vi "XY2.vi"() -> (3 "XY Graph":cluster{"X":dbl, "Y":dbl}[](graph))   [LabVIEW 2023]
panel:
  in  "error constant 2":errorcluster
  out "error constant":errorcluster
  in  "XY Graph 2":cluster{"X":dbl, "Y":dbl}[](graph)
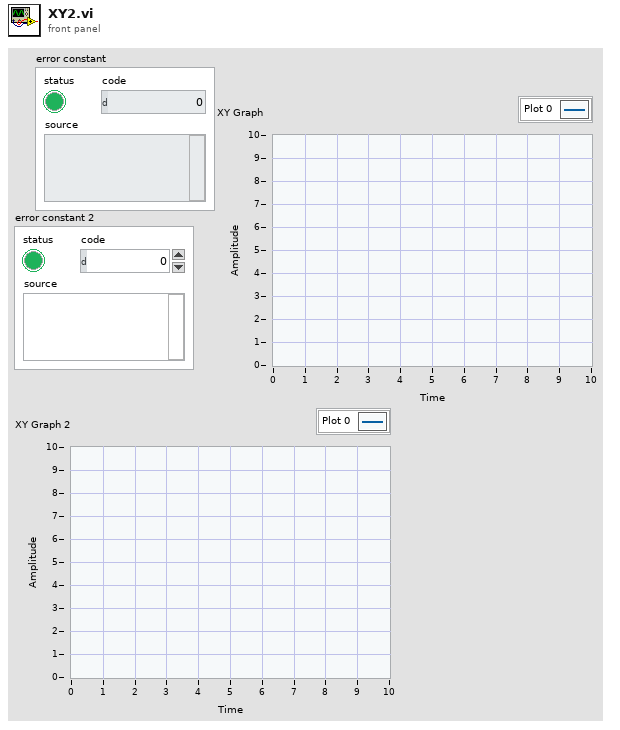
[diagram p1: front panel]
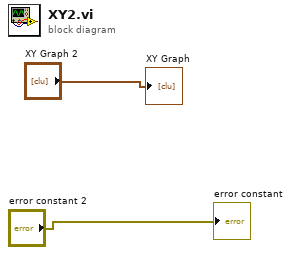
[diagram p0: block diagram]
diagram:
  "XY Graph" <- "XY Graph 2"
  "error constant" <- "error constant 2"
